vi "Get Capacitance.vi"(8 "error in (no error)":errorcluster, 9 "Channel":i32, 11 "AH2500A in":refnum<class "AH2500A.lvclass">) -> (0 "error out":errorcluster, 2 "Capacitance (pF)":dbl, 3 "AH2500A out":refnum<class "AH2500A.lvclass">)   [LabVIEW 2019, in "AH2500A.lvclass"]
uses:
  AH2500A.lvclass
  C:/Program Files (x86)/National Instruments/LabVIEW 2019/user.lib/LevyLab/Instrument Framework/SMOs/Instrument/Instrument.lvclass
  <userlib>/LevyLab/Instrument Framework/SMOs/Instrument/Instrument.lvclass/Instrument.ctl
  AH2500A.lvclass/AH2500A.ctl
  <userlib>/LevyLab/Instrument Framework/SMOs/Instrument/Instrument.lvclass
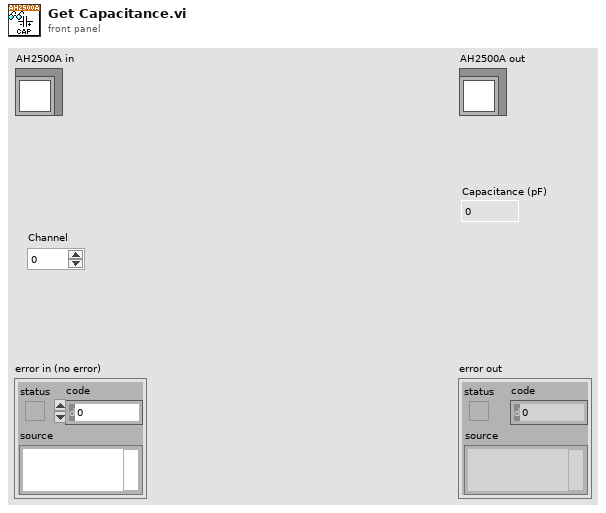
[diagram p1: front panel]
types:
  T1 = typedef "AH2500A.lvclass/AH2500A Measurement--Cluster.ctl" = cluster{"capacitance (pF)":dbl, "loss (nS)":dbl, "Vexc (V)":dbl}
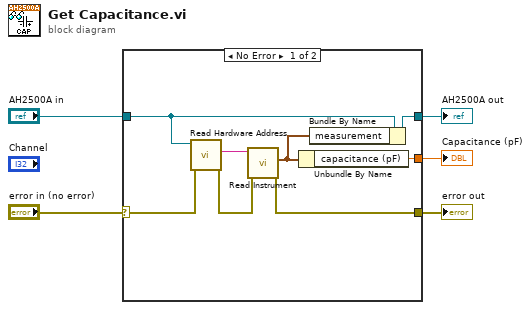
[diagram p0: block diagram]
diagram:
  n1 = case shown="No Error" "error in (no error)" {
    selector: "error in (no error)" -> [w12 w15]
    tunnel: [w11 w15] -> w4
    tunnel: [w8 w14] -> w3
    tunnel: [w9 _] -> w2
    tunnel: "AH2500A in" -> [w7 w14]
    frame No Error {
      n2 = call <userlib>:"Read Hardware Address.vi"("error in (no error)"=w12, "Instrument in"=w7) -> ("error out"=w10:errorcluster, "Address"=w13:string)  [unwired: 7 in, 1 out]
      n3 = call "Read Instrument.vi"("error in (no error)"=w10, "VISA resource name"=w13) -> ("error out"=w11:errorcluster, "Measurement"=w6:T1)  [unwired: 7 in, 1 out]
      n4 = Unbundle By Name(w6) -> ("capacitance (pF)"=w9:dbl)
      n5 = Bundle By Name(cluster=w7, "measurement"=w6) -> (w8:refnum<class "AH2500A.lvclass">)
    }
    frame Error {
    }
  }
  "error out" <- w4
  "AH2500A out" <- w3
  "Capacitance (pF)" <- w2
